vi "Main.vi"(8 "error in":errorcluster, 11 "Second Level Worker in":refnum<class "Second Level Worker.lvclass">) -> (0 "error out":errorcluster, 3 "Second Level Worker out":refnum<class "Second Level Worker.lvclass">)   [LabVIEW 2017, in "Method 2.lvlib" / "Second Level Worker.lvclass"]
doc: "The <b>Queued Message Handler</b> of the Worker that owns this VI."
uses:
  Second Level Worker.lvclass
  C:/Program Files (x86)/National Instruments/LabVIEW 2017/vi.lib/addons/_Workers/Library/Classes/Worker/Worker.lvclass
  Initialization Data.ctl
  Response Cases.ctl
  Second Level Worker.lvclass/Second Level Worker.ctl
  rql_Send Error to Caller.ctl
  <vilib>/addons/_Workers/Library/Classes/Message Queue/Message Queue.lvclass
panel:
  in  "Send Error to Caller":bool
  in  "User Error":errorcluster={"status"=TRUE, "code"=12345, "source"="Hello World! This is an error message."}
  # "Method 2 : Using the Workers Palette \"Send Error to Owner\" VI"
  # "Second Level Worker (Main VI)"
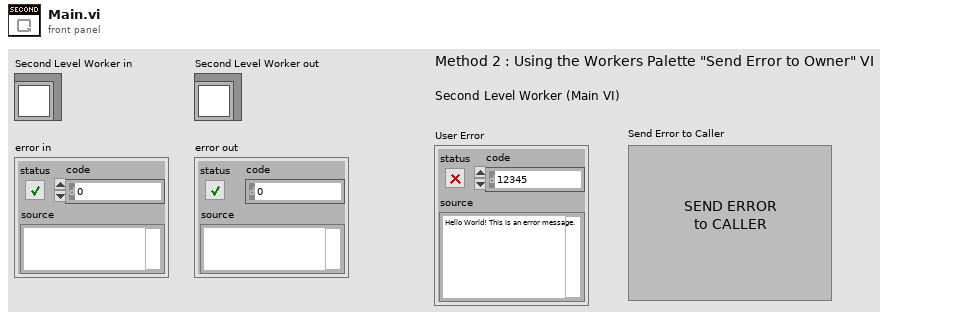
[diagram p1: front panel]
types:
  T1 = typedef "Method 2.lvlib/Second Level Worker.lvclass/Initialization Data.ctl" = cluster{"Response Cases":T2}
  T2 = typedef "Method 2.lvlib/Second Level Worker.lvclass/Response Cases.ctl" = cluster{"Placeholder - Can be deleted":string}
  T3 = typedef "Method 2.lvlib/Second Level Worker.lvclass/rql_Send Error to Caller.ctl" = cluster{"String":string}
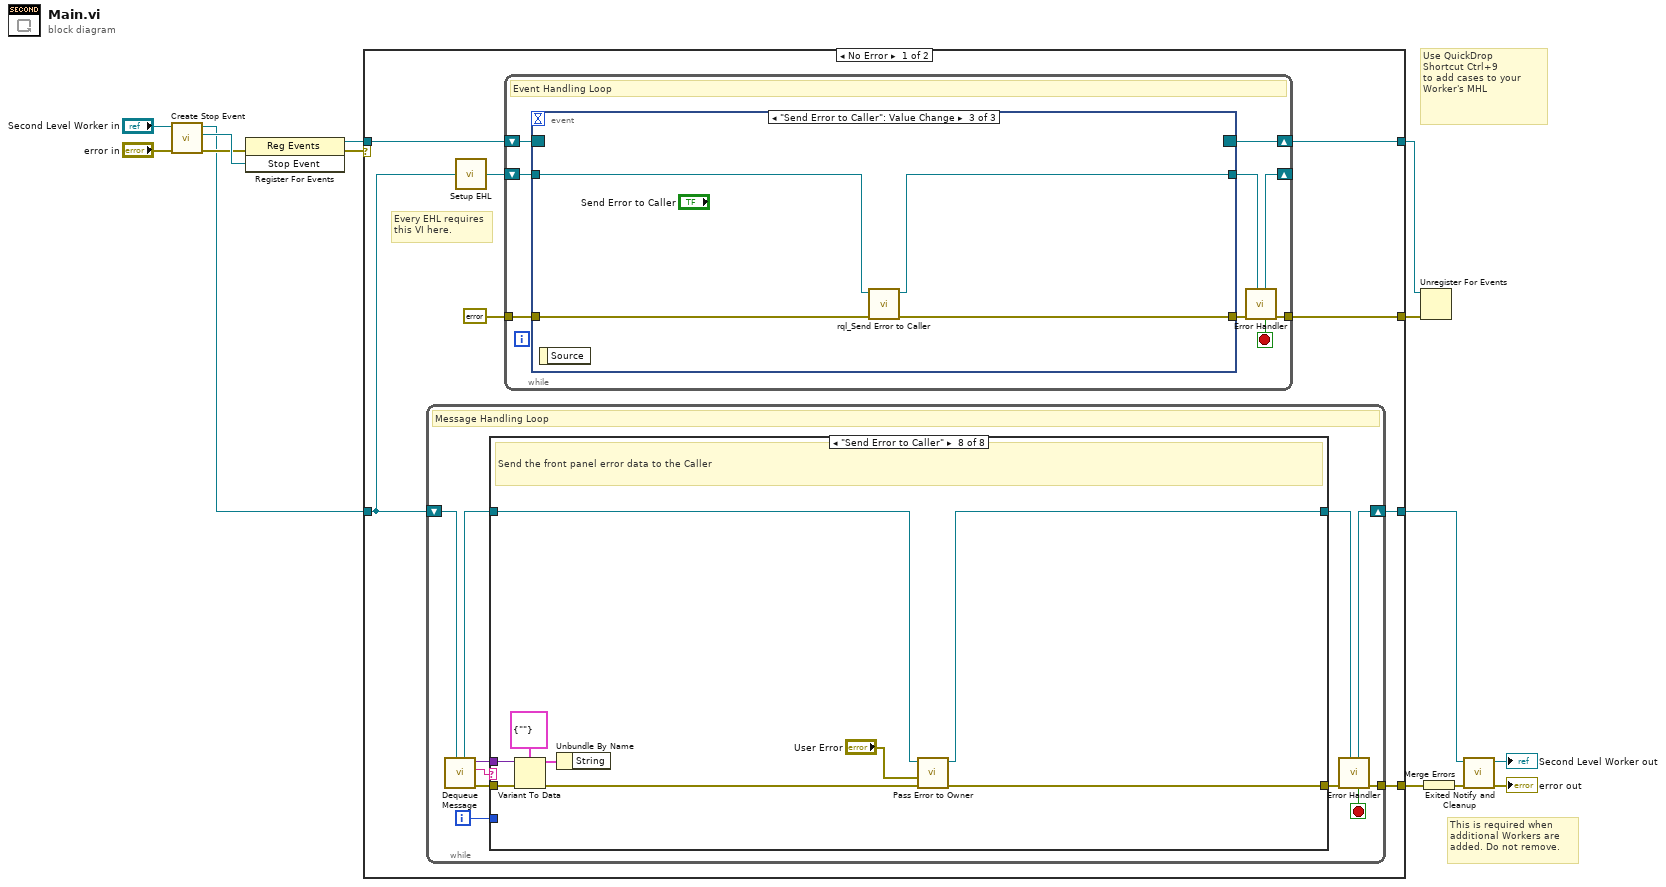
[diagram p0: block diagram]
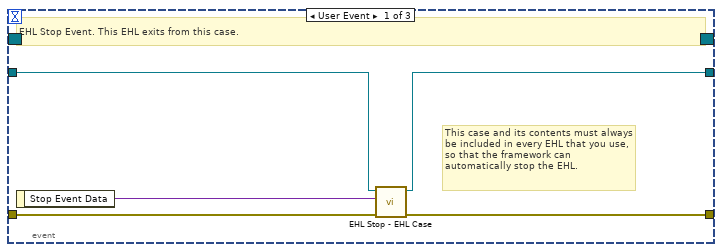
[diagram p2: hidden frame]
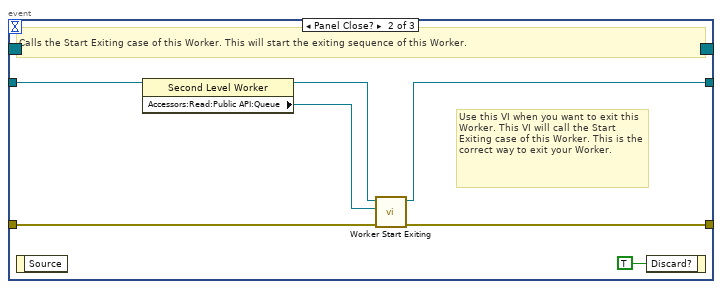
[diagram p3: hidden frame]
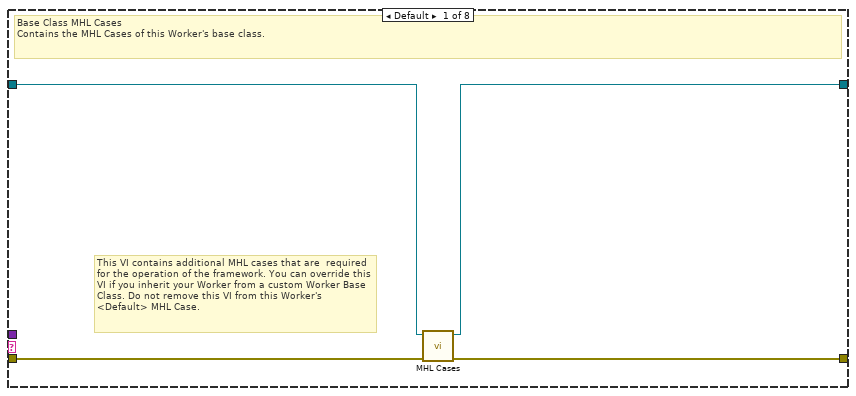
[diagram p4: hidden frame]
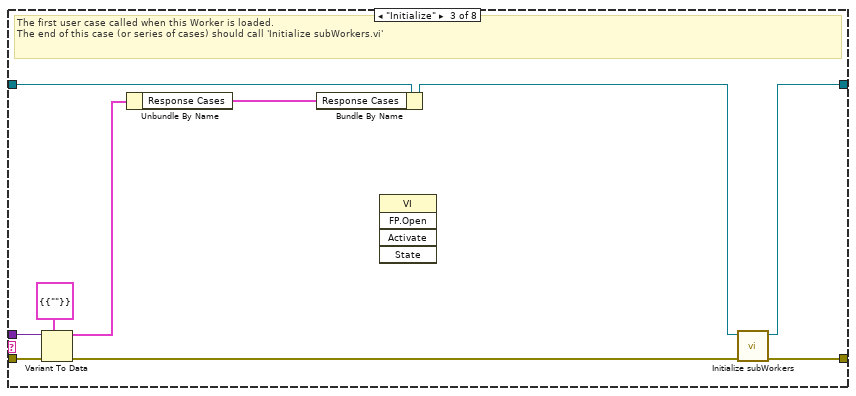
[diagram p6: hidden frame]
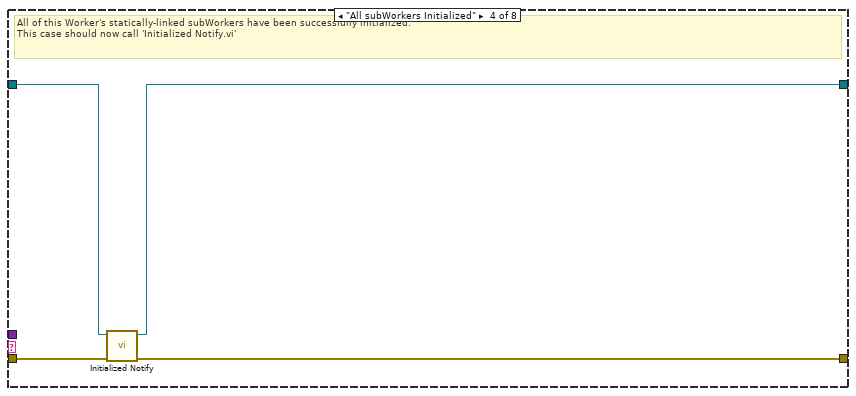
[diagram p7: hidden frame]
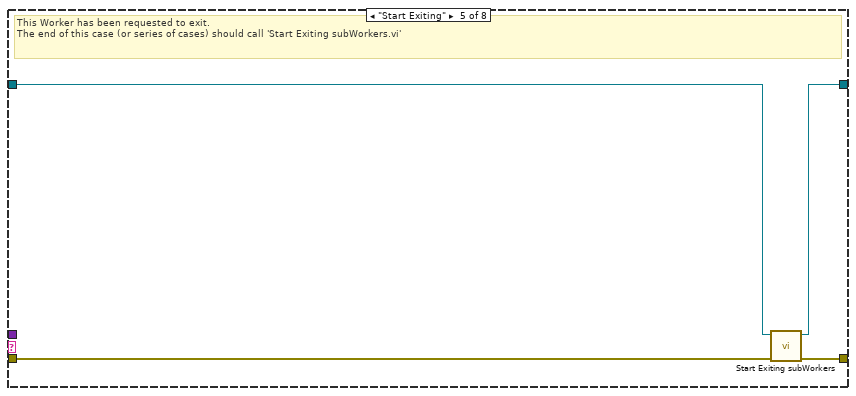
[diagram p8: hidden frame]
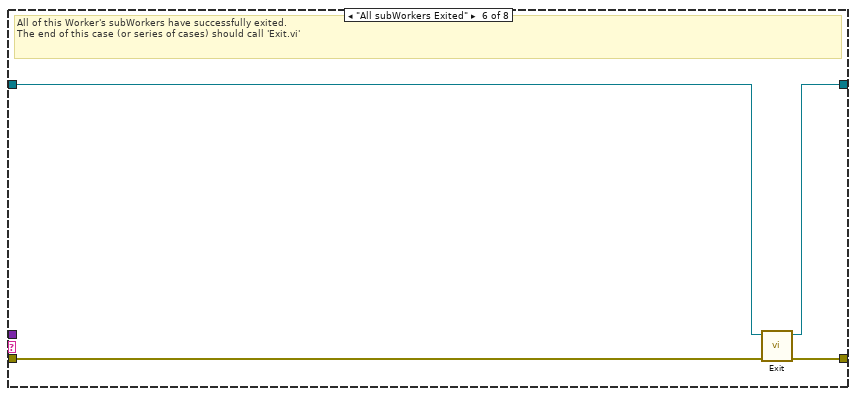
[diagram p9: hidden frame]
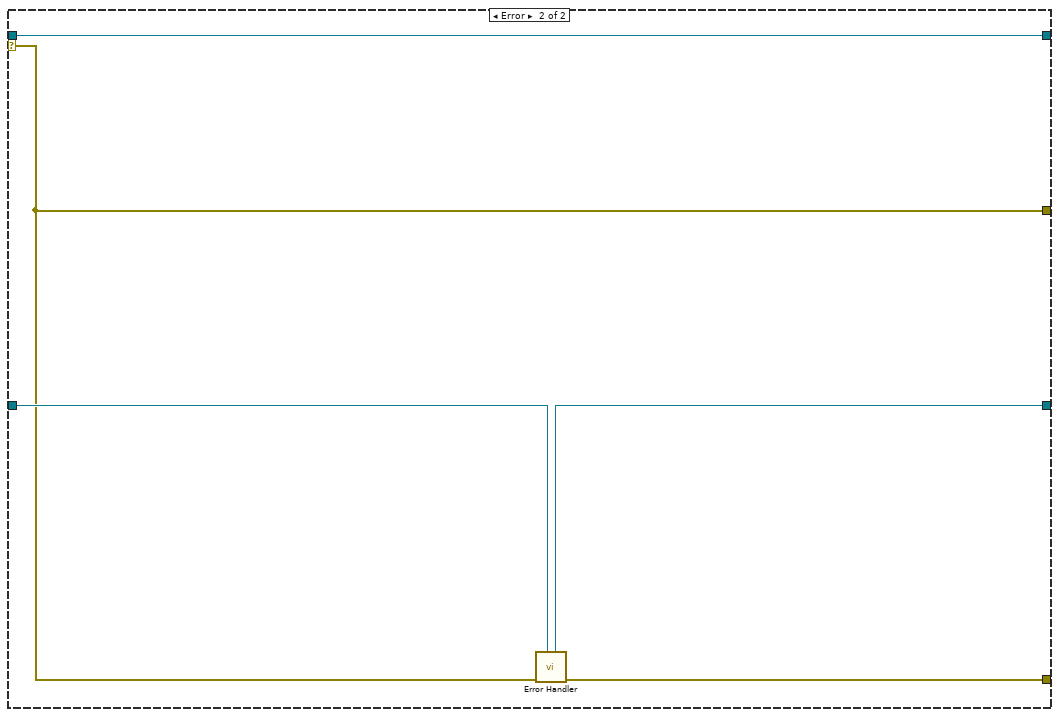
[diagram p11: hidden frame]
diagram:
  # "Use QuickDrop\nShortcut Ctrl+9\nto add cases to your\nWorker's MHL"
  # "This is required when additional Workers are added. Do not remove."
  n1 = call-dynamic "Create Stop Event.vi"("error in"="error in", "Worker"="Second Level Worker in") -> ("error out"=w6:errorcluster, "Stop Event"=w7:refnum<user-event>, "Worker out"=w3:refnum<class "Second Level Worker.lvclass">)  [unwired: 7 in]
  n2 = register-events(error in=w6, w7) -> (reference out=w5:refnum<event-registration>, error out=w4:errorcluster)  [unwired: 1 in]
  n3 = case shown="No Error" w4 {
    tunnel: w3 -> [w16 w101]
    tunnel: [w22 w102] -> w13
    tunnel: [w21 w100] -> w14
    selector: w4 -> [_ w99]
    tunnel: [w18 w98] -> w9
    tunnel: [w17 w99] -> w8
    tunnel: w5 -> [w15 w98]
    frame No Error {
      # "Every EHL requires\nthis VI here."
      n4 = while {
        shift-right: [w56] -> w21
        shift-left: w16 -> [w58]
        tunnel: [w57] -> w22
        i -> [w49]
        stop <- w50 stop-if-true
        # "Message Handling Loop"
        n5 = call-dynamic "Dequeue Message.vi"("Worker"=w58) -> ("error out"=w55:errorcluster, "Case out"=w51:string, "Data out"=w48:variant, "Worker out"=w53:refnum<class "Second Level Worker.lvclass">)  [unwired: 6 in, 1 out]
        n6 = case "Worker MHL Case Structure (DO NOT CHANGE LABEL NAME)" shown="\"Send Error to Caller\"" w51 {
          tunnel: w55 -> [w62 w63 w72 w78 w79 w86 w88 w97]
          tunnel: [w61 w63 w74 w77 w82 w85 w88 w93] -> w54
          tunnel: w53 -> [w60 w64 w71 w76 w80 w84 w87 w92]
          tunnel: [w59 w64 w73 w75 w81 w83 w87 w91] -> w52
          tunnel: w49 -> [_ _ _ _ _ _ _ _]
          tunnel: w48 -> [_ _ w69 _ _ _ _ w95]
          frame Default {
            # "This VI contains additional MHL cases that are  required for the operation of the framework. You can override this VI if you inherit your Worker from a custom Worker Base Class. Do not remove this VI from this Worker's <Default> MHL Case."
            # "Base Class MHL Cases\nContains the MHL Cases of this Worker's base class."
            n7 = call-dynamic "MHL Cases.vi"("error in"=w62, "Worker in"=w60) -> ("error out"=w61:errorcluster, "Worker out"=w59:refnum<class "Second Level Worker.lvclass">)  [unwired: 8 in]
          }
          frame "------------ FRAMEWORK CASES -----------" {
            # "Start of Workers Framework Cases"
          }
          frame "Initialize" {
            # "The first user case called when this Worker is loaded.\nThe end of this case (or series of cases) should call 'Initialize subWorkers.vi'"
            n8 = Variant To Data(error in=w72, type=T1 {"Response Cases"={"Placeholder - Can be deleted"=""}} ("Cluster"), Variant=w69) -> (data=w67:T1, error out=w70:errorcluster)
            n9 = Unbundle By Name(w67) -> ("Response Cases"=w66:T2)
            n10 = Bundle By Name(cluster=w71, "Response Cases"=w66) -> (w68:refnum<class "Second Level Worker.lvclass">)
            n11 = invoke class="VI" method="FP.Open"() -> ()  [unwired: 5 in, 5 out]
            n12 = call-dynamic "Initialize subWorkers.vi"("error in"=w70, "Worker"=w68) -> ("error out"=w74:errorcluster, "dup Worker out"=w73:refnum<class "Second Level Worker.lvclass">)  [unwired: 8 in]
          }
          frame "All subWorkers Initialized" {
            # "All of this Worker's statically-linked subWorkers have been successfully initialized.\nThis case should now call 'Initialized Notify.vi'"
            n13 = call-dynamic "Initialized Notify.vi"("error in"=w78, "Worker"=w76) -> ("error out"=w77:errorcluster, "dup Worker out"=w75:refnum<class "Second Level Worker.lvclass">)  [unwired: 8 in]
          }
          frame "Start Exiting" {
            # "This Worker has been requested to exit. \nThe end of this case (or series of cases) should call 'Start Exiting subWorkers.vi'"
            n14 = call-dynamic "Start Exiting subWorkers.vi"("error_in"=w79, "Worker"=w80) -> ("error out"=w82:errorcluster, "dup Worker out"=w81:refnum<class "Second Level Worker.lvclass">)  [unwired: 8 in]
          }
          frame "All subWorkers Exited" {
            # "All of this Worker's subWorkers have successfully exited. \nThe end of this case (or series of cases) should call 'Exit.vi'"
            n15 = call-dynamic "Exit.vi"("error_in"=w86, "Worker"=w84) -> ("error out"=w85:errorcluster, "dup Worker out"=w83:refnum<class "Second Level Worker.lvclass">)  [unwired: 8 in]
          }
          frame "------------- LOCAL API CASES -------------" {
            # "Start of Workers Local API Cases"
          }
          frame "Send Error to Caller" {
            # "Send the front panel error data to the Caller"
            n16 = Variant To Data(error in=w97, type=T3 {"String"=""} ("Data"), Variant=w95) -> (data=w94:T3, error out=w90:errorcluster)
            n17 = Unbundle By Name(w94) -> ()  [unwired: 1 out]
            n18 = call-dynamic "Pass Error to Owner.vi"("error_in"=w90, "Error to Pass to Owner"="User Error", "Worker"=w92) -> ("error out"=w93:errorcluster, "dup Worker out"=w91:refnum<class "Second Level Worker.lvclass">)  [unwired: 7 in]
          }
        }
        n19 = call-dynamic "Error Handler.vi"("Worker"=w52, "error_in"=w54) -> ("error out"=w57:errorcluster, "Stop Loop"=w50:bool, "Worker out"=w56:refnum<class "Second Level Worker.lvclass">)  [unwired: 7 in]
      }
      n20 = call-dynamic "Setup EHL.vi"("Worker"=w16) -> ("Worker out"=w19:refnum<class "Second Level Worker.lvclass">)  [unwired: 14 in]
      n21 = while "Event Handling Loop" {
        shift-right: [w31] -> w18
        shift-left: w15 -> [w30]
        tunnel: [w26] -> w17
        tunnel: errorcluster {"status"=FALSE, "code"=0, "source"=""} ("error constant") -> [w28]
        shift-right: [w24] -> _
        shift-left: w19 -> [w29]
        stop <- w23 stop-if-true
        # "Event Handling Loop"
        n22 = event shown="[2] \"Send Error to Caller\": Value Change" {
          selector: w30 -> [_ _ _]
          dyn-events: [_ _ _] -> w31
          timeout: _ -> [_ _ _]
          tunnel: [w35 w42 w46] -> w27
          tunnel: w28 -> [w36 w41 w47]
          tunnel: w29 -> [w34 w40 w45]
          tunnel: [w33 w39 w44] -> w25
          event User Event {
            # "This case and its contents must always be included in every EHL that you use, so that the framework can automatically stop the EHL."
            # "EHL Stop Event. This EHL exits from this case."
            n23 = event-data() -> ("Stop Event Data"=w32:variant)  [unwired: 1 in]
            n24 = call-dynamic "EHL Stop - EHL Case.vi"("error in"=w36, "Stop Event Data"=w32, "Worker"=w34) -> ("error out"=w35:errorcluster, "Worker out"=w33:refnum<class "Second Level Worker.lvclass">)  [unwired: 7 in]
          }
          event Panel Close? {
            # "Use this VI when you want to exit this Worker. This VI will call the Start Exiting case of this Worker. This is the correct way to exit your Worker."
            # "Calls the Start Exiting case of this Worker. This will start the exiting sequence of this Worker."
            n25 = event-data() -> ()  [unwired: 1 in, 1 out]
            n26 = property class="Second Level Worker"(reference=w40) -> (reference out=w38:refnum<class "Second Level Worker.lvclass">, "Accessors:Read:Public API:Queue"=w37:refnum<class "Message Queue.lvclass">)  [unwired: 1 in, 1 out]
            n27 = call-dynamic "Worker Start Exiting.vi"("error_in"=w41, "Message Queue"=w37, "Worker"=w38) -> ("error out"=w42:errorcluster, "dup Worker out"=w39:refnum<class "Second Level Worker.lvclass">)  [unwired: 7 in]
            n28 = event-data ("Event Filter Node")("Discard?"=TRUE) -> ()  [unwired: 1 in, 1 out]
          }
          event "Send Error to Caller": Value Change {
            n29 = event-data() -> ()  [unwired: 1 in, 1 out]
            n30 = call "rql_Send Error to Caller.vi"("error in"=w47, "Second Level Worker in"=w45) -> ("error out"=w46:errorcluster, "dup Second Level Worker out"=w44:refnum<class "Second Level Worker.lvclass">)  [unwired: 8 in]
          }
        }
        n31 = call-dynamic "Error Handler.vi"("Worker"=w25, "error_in"=w27) -> ("error out"=w26:errorcluster, "Stop Loop"=w23:bool, "Worker out"=w24:refnum<class "Second Level Worker.lvclass">)  [unwired: 7 in]
      }
    }
    frame Error {
      n32 = call-dynamic "Error Handler.vi"("Worker"=w101, "error_in"=w99) -> ("error out"=w102:errorcluster, "Worker out"=w100:refnum<class "Second Level Worker.lvclass">)  [unwired: 7 in, 1 out]
    }
  }
  n33 = Unregister For Events(event registration refnum=w9, error in=w8) -> ()  [unwired: 1 out]
  n34 = Merge Errors(w13) -> (w10:errorcluster)
  n35 = call-dynamic "Exited Notify and Cleanup.vi"("error_in"=w10, "Worker"=w14) -> ("error out"=→"error out":errorcluster, "dup Worker out"=→"Second Level Worker out":refnum<class "Second Level Worker.lvclass">)  [unwired: 8 in]
